vi "TerminationChecker.vi"(10 "Type":T1(ring)=enum."LineFeed", 11 "input string":string) -> (3 "Ret":bool)   [LabVIEW 2017]
panel:
  out "substring":string
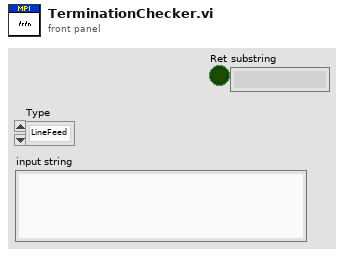
[diagram p1: front panel]
types:
  T1 = enum16{"EndOfLine", "LineFeed", "CarriageReturn"}
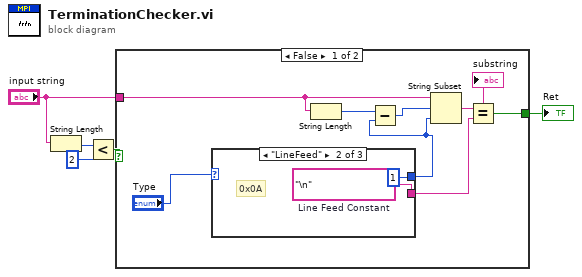
[diagram p0: block diagram]
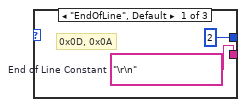
[diagram p2: hidden frame]
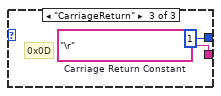
[diagram p3: hidden frame]
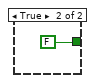
[diagram p4: hidden frame]
diagram:
  n1 = String Length(string="input string") -> (length=w2:i32)
  n2 = Less?(x=w2, y=2) -> (x < y?=w3:bool)
  n3 = case shown="False" w3 {
    tunnel: [w10 FALSE] -> w5
    tunnel: "input string" -> [w8 _]
    frame False {
      n4 = case shown="\"LineFeed\"" "Type" {
        tunnel: [w15 w17 w19] -> w9
        tunnel: [2 1 1] -> w6
        frame "EndOfLine", Default {
          w15 = "\r\n"  # End of Line Constant
          # "0x0D, 0x0A"
        }
        frame "LineFeed" {
          w17 = "\n"  # Line Feed Constant
          # "0x0A"
        }
        frame "CarriageReturn" {
          w19 = "\r"  # Carriage Return Constant
          # "0x0D"
        }
      }
      n5 = String Length(string=w8) -> (length=w11:i32)
      n6 = Subtract(x=w11, y=w6) -> (x-y=w13:i32)
      n7 = String Subset(string=w8, offset (0)=w13, length (rest)=w6) -> (substring=w12:string)
      "substring" <- w12
      n8 = Equal?(x=w12, y=w9) -> (x = y?=w10:bool)
    }
    frame True {
    }
  }
  "Ret" <- w5
